vi "Instrument Get Private.vi"(1 "Variant":variant) -> (0 "Private":T1 {"Offset" format="%^_3e"; "Scale Factors" format="%^_3e"})   [LabVIEW 2025]
doc: "Author: Scott Hannahs <sth@magnet.fsu.edu>\n\nThis software is licensed for use under the “MIT License\"\nCopyright (c) 2025 Scott Hannahs, sth@sth@magnet.sthnet.net\n\nPermission is hereby granted, free of charge, to any person obtaining a copy of this software and associated documentation files (the \"Software\"), to deal in the Software without restriction, including without limitation the rights to use, copy, modify, merge, publish, distribute, sublicense, and/or sell copies of the Software, and to permit persons to whom the Software is furnished to do so, subject to the following conditions: The above copyright notice and this permission notice shall be included in all copies or substantial portions of the Software.\n\nTHE SOFTWARE IS PROVIDED \"AS IS\", WITHOUT WARRANTY OF ANY KIND, EXPRESS OR IMPLIED, INCLUDING BUT NOT LIMITED TO THE WARRANTIES OF MERCHANTABILITY, FITNESS FOR A PARTICULAR PURPOSE AND NONINFRINGEMENT. IN NO EVENT SHALL THE AUTHORS OR COPYRIGHT HOLDERS BE LIABLE FOR ANY CLAIM, DAMAGES OR OTHER LIABILITY, WHETHER IN AN ACTION OF CONTRACT, TORT OR OTHERWISE, ARISING FROM, OUT OF OR IN CONNECTION WITH THE SOFTWARE OR THE USE OR OTHER DEALINGS IN THE SOFTWARE."
uses:
  Sub Controls/Private.ctl
  Sub Controls/Instrument Ref.ctl
  Sub Controls/SystemCheckBox-resize.ctl
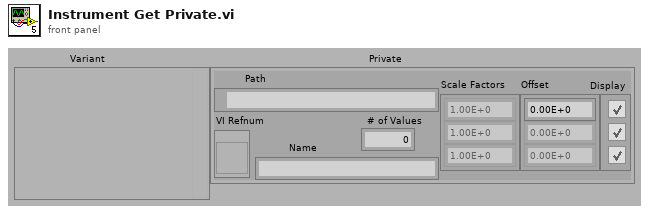
[diagram p1: front panel]
types:
  T1 = typedef "Private.ctl" = cluster{"Path":path, "VI Refnum":T2, "Name":string, "# of Values":i32, "Scale Factors":dbl[], "Display":T3[], "Offset":dbl[]}
  T2 = typedef "Instrument Ref.ctl" = refnum<vi>
  T3 = typedef "SystemCheckBox-resize.ctl" = bool
  T4 = typedef "Instrument Properties.ctl" = cluster{"Public":T5, "Private":T1}
  T5 = typedef "Public.ctl" = cluster{"Column Name":string[], "Trace Color":u32[]}
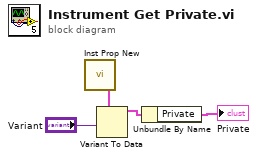
[diagram p0: block diagram]
diagram:
  n1 = call "Inst Prop New.vi"() -> ("Instrument Prop Out"=w3:T4)
  n2 = Variant To Data(type=w3, Variant="Variant") -> (data=w1:T4)  [unwired: 1 in, 1 out]
  n3 = Unbundle By Name(w1) -> ("Private"=→"Private":T1)
